vi "Decide Whether To Show The Error Window.vi"(8 "Error In":errorcluster, 9 "Show Error Window (Default Setting)":T1, 10 "Newly Reported Error":T2, 11 "Module Data in":T4) -> (0 "Error Out":errorcluster)   [LabVIEW 2023, in "Error Manager.lvlib"]
doc: "This VI decides whether the <B>Error Window</B> should be popped-up (displayed) to the user."
uses:
  Error Manager.lvlib
  Module Data (cluster).ctl
  GUI Object References (cluster).ctl
  Handled Error (cluster).ctl
  Read-Unread Status (enum).ctl
  Display Order (enum).ctl
  Error in current one-second interval (cluster).ctl
  Reported Error (cluster).ctl
  Public API VIs/Show Error Window Instruction (enum).ctl
  Settings/Show_Error_Window_Default (enum).ctl
  Queues/New Error Window Loop Queue/Error Window Loop Queue.lvclass
  Settings/Settings.lvclass
panel:
  out "Show the Error Window?":bool
  # "Development\nControls or indicators that are useful for development or testing, but which are not outputs of the VI."
  # "Input\nInputs to the VI"
  # "Output\nOutputs of the VI"
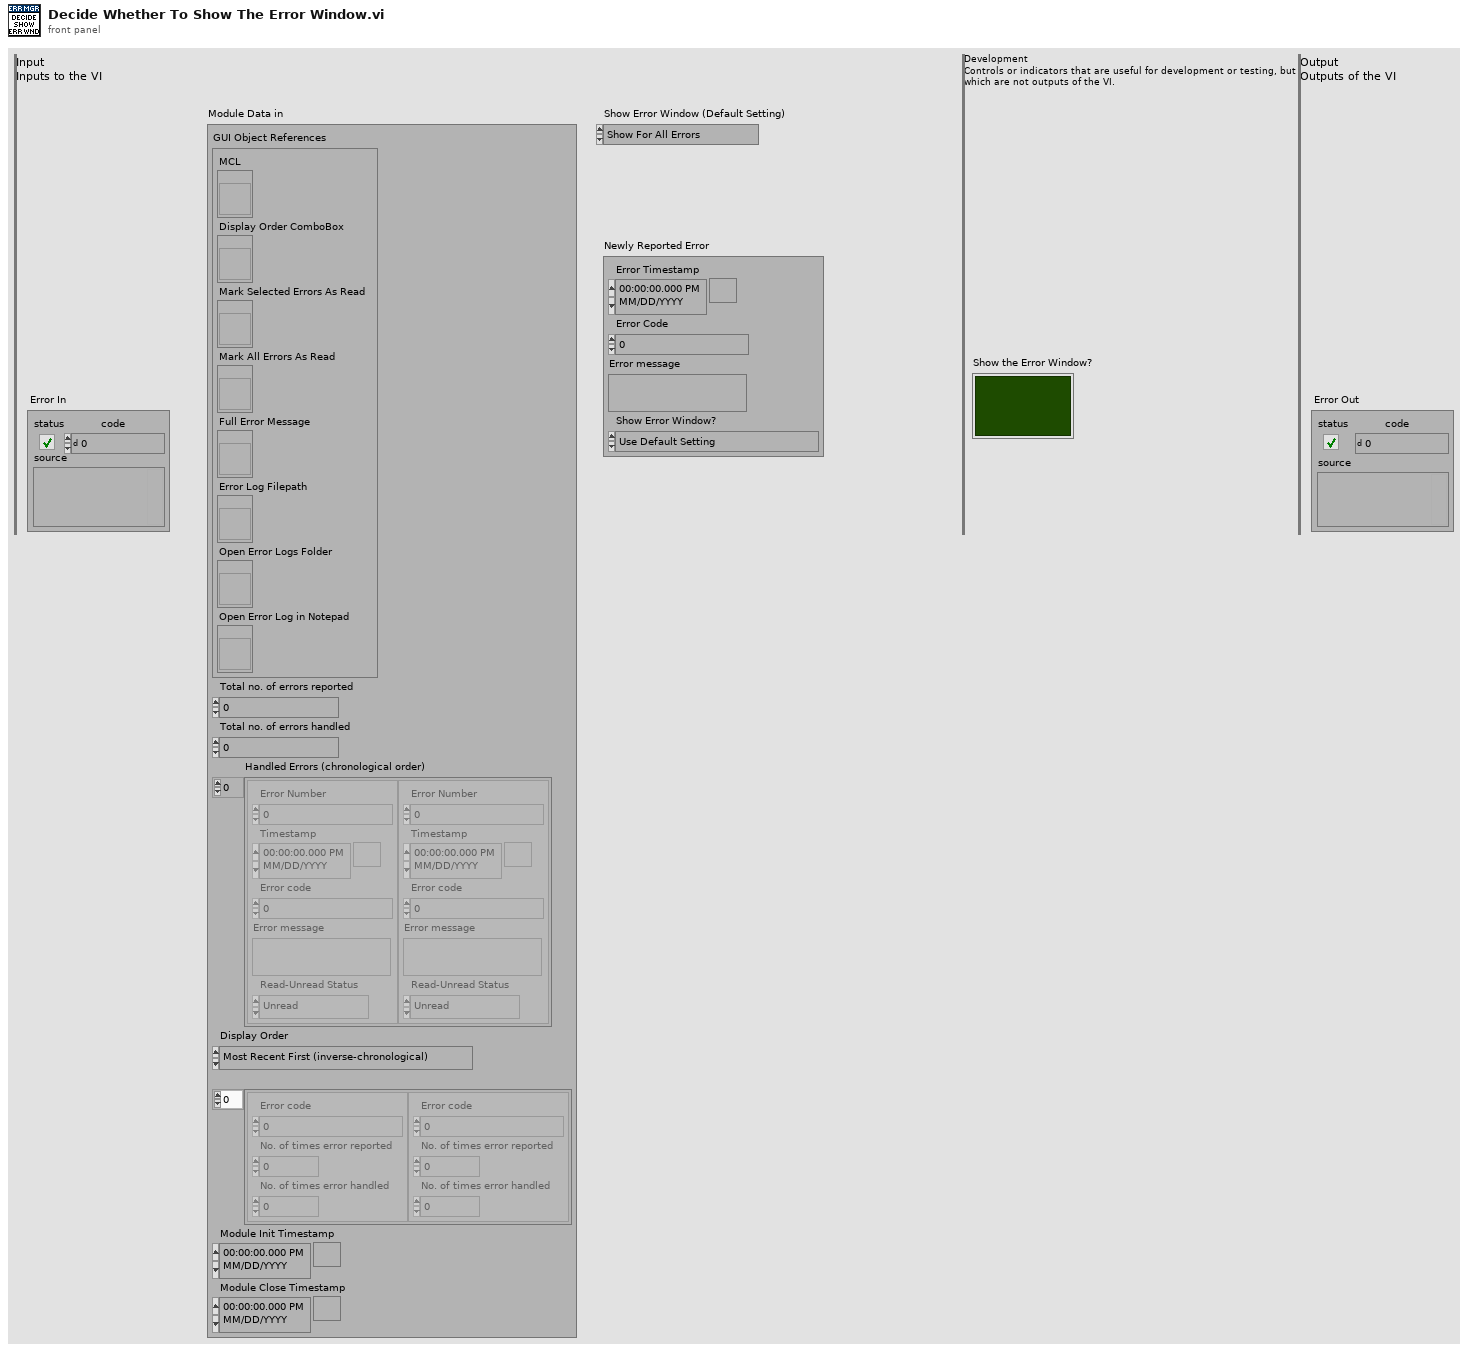
[diagram p1: front panel]
types:
  T1 = typedef "Error Manager.lvlib/Settings.lvclass/Show_Error_Window_Default (enum).ctl" = enum16{"Show For All Errors", "Show For New Errors", "Show For New Error Codes", "Do Not Show"}
  T2 = typedef "Error Manager.lvlib/Reported Error (cluster).ctl" = cluster{"Error Timestamp":timestamp, "Error Code":i32, "Error message":string, "Show Error Window?":T3}
  T3 = typedef "Error Manager.lvlib/Show Error Window Instruction (enum).ctl" = enum16{"Use Default Setting", "Show", "Do Not Show"}
  T4 = typedef "Error Manager.lvlib/Module Data (cluster).ctl" = cluster{"GUI Object References":T5, "Total no. of errors reported":i32, "Total no. of errors handled":i32, "Handled Errors (chronological order)":T6[], "Display Order":T8, "Errors in current one-second interval":T9[], "Module Init Timestamp":timestamp, "Module Close Timestamp":timestamp}
  T5 = typedef "Error Manager.lvlib/GUI Object References (cluster).ctl" = cluster{"MCL":refnum<vi>, "Display Order ComboBox":refnum<vi>, "Mark Selected Errors As Read":refnum<vi>, "Mark All Errors As Read":refnum<vi>, "Full Error Message":refnum<vi>, "Error Log Filepath":refnum<vi>, "Open Error Logs Folder":refnum<vi>, "Open Error Log in Notepad":refnum<vi>}
  T6 = typedef "Error Manager.lvlib/Handled Error (cluster).ctl" = cluster{"Error Number":i32, "Timestamp":timestamp, "Error code":i32, "Error message":string, "Read-Unread Status":T7}
  T7 = typedef "Error Manager.lvlib/Read-Unread Status (enum).ctl" = enum16{"Unread", "Read"}
  T8 = typedef "Error Manager.lvlib/Display Order (enum).ctl" = enum16{"Most Recent First (inverse-chronological)", "Oldest First (chronological)"}
  T9 = typedef "Error Manager.lvlib/Error in current one-second interval (cluster).ctl" = cluster{"Error code":i32, "No. of times error reported":u32, "No. of times error handled":u32}
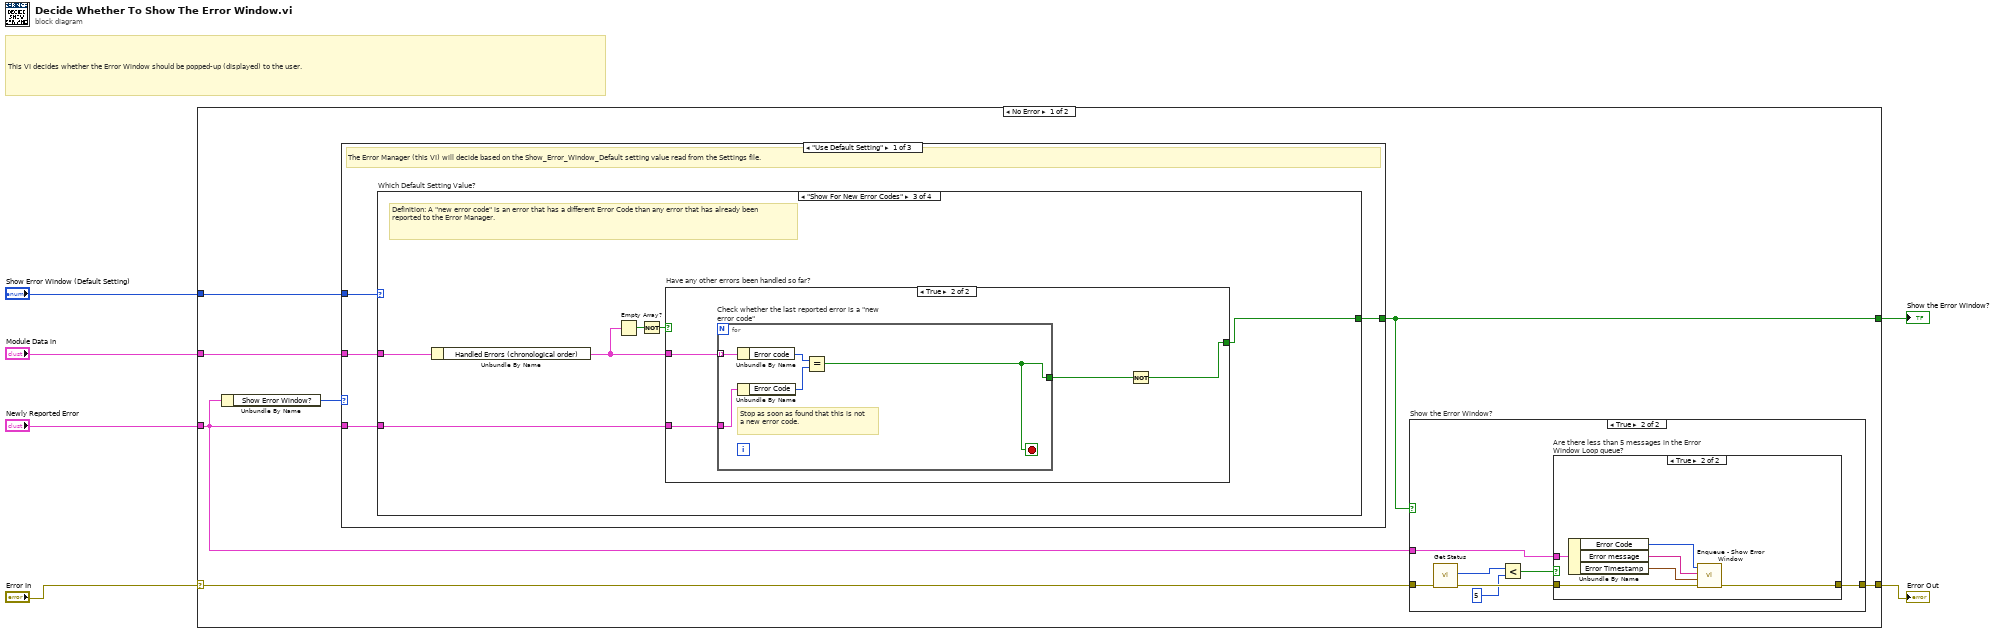
[diagram p0: block diagram]
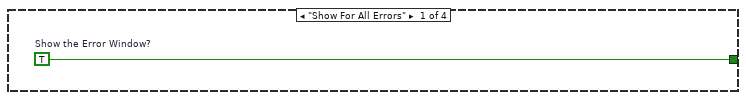
[diagram p2: hidden frame]
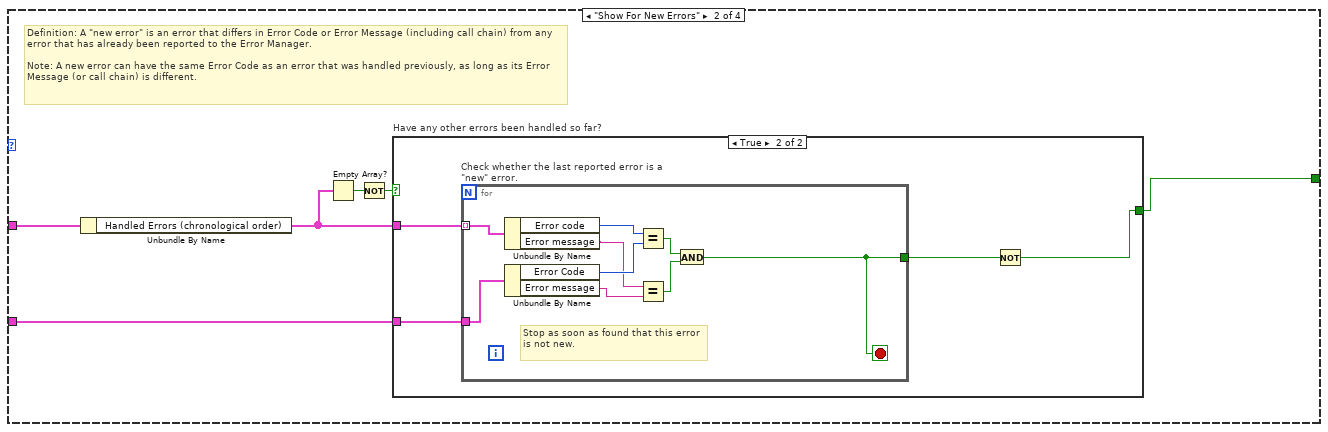
[diagram p3: hidden frame]
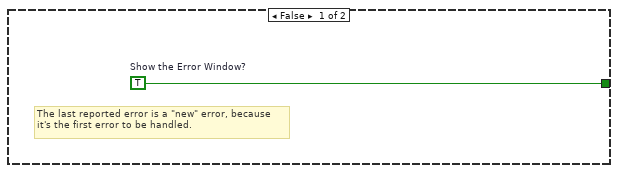
[diagram p4: hidden frame]
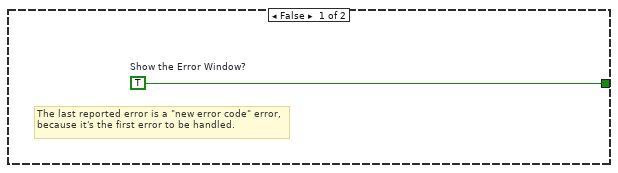
[diagram p5: hidden frame]
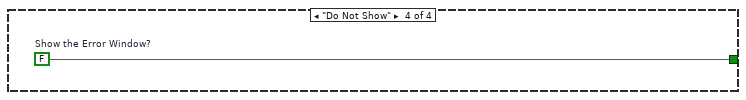
[diagram p6: hidden frame]
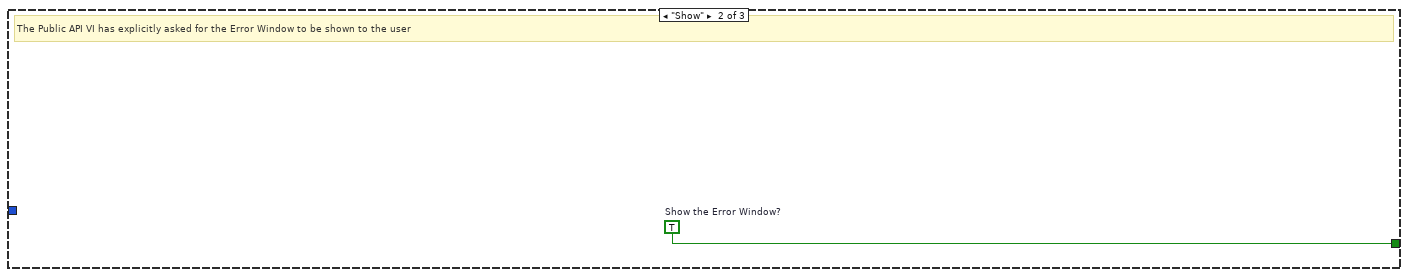
[diagram p7: hidden frame]
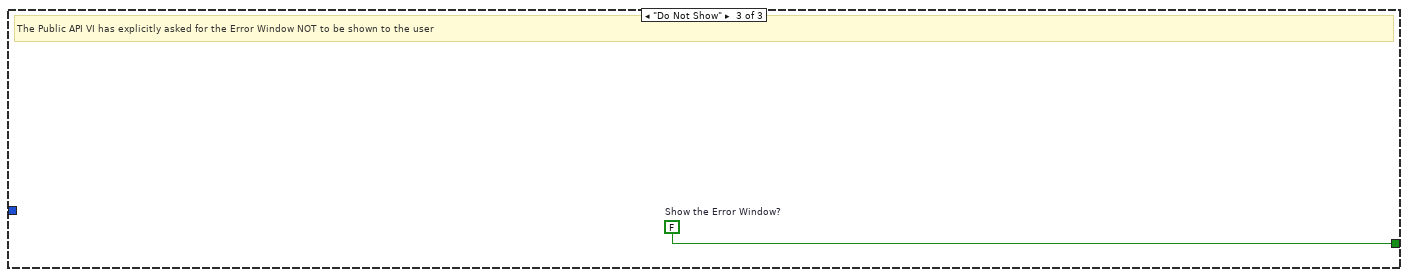
[diagram p8: hidden frame]
diagram:
  # "This VI decides whether the Error Window should be popped-up (displayed) to the user."
  n1 = case shown="No Error" "Error In" {
    selector: "Error In" -> [w11 w73]
    tunnel: [w10 w73] -> w5
    tunnel: "Module Data in" -> [w13 _]
    tunnel: "Newly Reported Error" -> [w9 _]
    tunnel: "Show Error Window (Default Setting)" -> [w12 _]
    tunnel: [w7 _] -> w1
    frame No Error {
      n2 = Unbundle By Name(w9) -> ("Show Error Window?"=w8:T3)
      n3 = case shown="\"Use Default Setting\"" w8 {
        tunnel: w13 -> [w17 _ _]
        tunnel: w12 -> [w16 _ _]
        tunnel: [w15 w56 w57] -> w7
        tunnel: w9 -> [w14 _ _]
        frame "Use Default Setting" {
          # "The Error Manager (this VI) will decide based on the Show_Error_Window_Default setting value read from the Settings file."
          n4 = case "Which Default Setting Value?" shown="\"Show For New Error Codes\"" w16 {
            tunnel: w17 -> [_ w24 w44 _]
            tunnel: w14 -> [_ w23 w43 _]
            tunnel: [w18 w22 w42 w55] -> w15
            frame "Show For All Errors" {
              w18 = TRUE  # Show the Error Window?
            }
            frame "Show For New Errors" {
              # "Definition: A \"new error\" is an error that differs in Error Code or Error Message (including call chain) from any error that has already been reported to the Error Manager.\n\nNote: A new error can have the same Error Code as an error that was handled previously, as long as its Error Message (or call chain) is different."
              n5 = Unbundle By Name(w24) -> ("Handled Errors (chronological order)"=w19:T6[])
              n6 = Empty Array?(array=w19) -> (empty?=w21:bool)
              n7 = Not(x=w21) -> (.not. x?=w20:bool)
              n8 = case "Have any other errors been handled so far?" shown="True" w20 {
                tunnel: [w25 w26] -> w22
                tunnel: w19 -> [_ w29]
                tunnel: w23 -> [_ w28]
                frame False {
                  w25 = TRUE  # Show the Error Window?
                  # "The last reported error is a \"new\" error, because it's the first error to be handled."
                }
                frame True {
                  n9 = for "Check whether the last reported error is a \"new\" error." {
                    tunnel: w29 -> [w37] mode=indexing
                    tunnel: w28 -> [w38]
                    tunnel: [w30] -> w27
                    stop <- w30 stop-if-true
                    # "Stop as soon as found that this error is not new."
                    n10 = Unbundle By Name(w37) -> ("Error code"=w36:i32, "Error message"=w34:string)
                    n11 = Unbundle By Name(w38) -> ("Error Code"=w35:i32, "Error message"=w33:string)
                    n12 = Equal?(x=w36, y=w35) -> (x = y?=w31:bool)
                    n13 = Equal?(x=w34, y=w33) -> (x = y?=w32:bool)
                    n14 = And(x=w31, y=w32) -> (x .and. y?=w30:bool)
                  }
                  n15 = Not(x=w27) -> (.not. x?=w26:bool)
                }
              }
            }
            frame "Show For New Error Codes" {
              # "Definition: A \"new error code\" is an error that has a different Error Code than any error that has already been reported to the Error Manager."
              n16 = Unbundle By Name(w44) -> ("Handled Errors (chronological order)"=w39:T6[])
              n17 = Empty Array?(array=w39) -> (empty?=w41:bool)
              n18 = Not(x=w41) -> (.not. x?=w40:bool)
              n19 = case "Have any other errors been handled so far?" shown="True" w40 {
                tunnel: [w45 w46] -> w42
                tunnel: w39 -> [_ w49]
                tunnel: w43 -> [_ w48]
                frame False {
                  w45 = TRUE  # Show the Error Window?
                  # "The last reported error is a \"new error code\" error, because it's the first error to be handled."
                }
                frame True {
                  n20 = for "Check whether the last reported error is a \"new error code\"" {
                    tunnel: w49 -> [w53] mode=indexing
                    tunnel: w48 -> [w54]
                    tunnel: [w50] -> w47
                    stop <- w50 stop-if-true
                    # "Stop as soon as found that this is not a new error code."
                    n21 = Unbundle By Name(w54) -> ("Error Code"=w51:i32)
                    n22 = Unbundle By Name(w53) -> ("Error code"=w52:i32)
                    n23 = Equal?(x=w52, y=w51) -> (x = y?=w50:bool)
                  }
                  n24 = Not(x=w47) -> (.not. x?=w46:bool)
                }
              }
            }
            frame "Do Not Show" {
              w55 = FALSE  # Show the Error Window?
            }
          }
        }
        frame "Show" {
          w56 = TRUE  # Show the Error Window?
          # "The Public API VI has explicitly asked for the Error Window to be shown to the user"
        }
        frame "Do Not Show" {
          w57 = FALSE  # Show the Error Window?
          # "The Public API VI has explicitly asked for the Error Window NOT to be shown to the user"
        }
      }
      n25 = case "Show the Error Window?" shown="True" w7 {
        tunnel: w11 -> [w58 w62]
        tunnel: [w58 w65] -> w10
        tunnel: w9 -> [_ w64]
        frame False {
        }
        frame True {
          n26 = call "Get Status.vi"("error in (no error)"=w62) -> ("error out"=w63:errorcluster, "No. Of Elements in Queue"=w61:i32)  [unwired: 8 in, 1 out]
          n27 = Less?(x=w61, y=5) -> (x < y?=w59:bool)
          n28 = case "Are there less than 5 messages in the Error Window Loop queue?" shown="True" w59 {
            tunnel: [w66 w72] -> w65
            tunnel: w64 -> [_ w71]
            tunnel: w63 -> [w66 w67]
            frame False {
              # "It is likely that the messages in the Error Window Loop queue are \"Show Error Window\" commands.\n\nDo not enqueue another such command, as it could lead to the user having to press \"OK\" on too many consecutive windows."
            }
            frame True {
              n29 = Unbundle By Name(w71) -> ("Error Code"=w70:i32, "Error message"=w69:string, "Error Timestamp"=w68:timestamp)
              n30 = call "Enqueue - Show Error Window.vi"("Error In"=w67, "Error Timestamp"=w68, "Error Message"=w69, "Error Code"=w70) -> ("Error Out"=w72:errorcluster)  [unwired: 7 in]
            }
          }
        }
      }
    }
    frame Error {
    }
  }
  "Error Out" <- w5
  "Show the Error Window?" <- w1
